vi "Calculate Driving Direction of Tank2_0713.vi"(8 "error in (no error)":errorcluster, 10 "obstacle angles (rad)":dbl[](array[numeric]), 11 "obstacle distances (m)":dbl[](array[numeric])) -> (0 "error out":errorcluster, 3 "steering frame velocity":dbl[](array[numeric]))   [LabVIEW 2012]
doc: "Calculates the velocity vector of the robot required to avoid obstacles, based on the scanned data."
uses:
  <vilib>/robotics/Obstacle Avoidance/Simple Vector Field Histogram/Panic Range.ctl
  <vilib>/Utility/AngleManip/Degrees to Radians (Scalar DBL).vi
  <vilib>/robotics/Obstacle Avoidance/Simple Vector Field Histogram/NI_Robotics_Simple Vector Field Histogram.lvlib
  <vilib>/Utility/AngleManip/NI_AngleManipulation.lvlib
panel:
  out "steering frame velocity 2":dbl[](array[numeric])
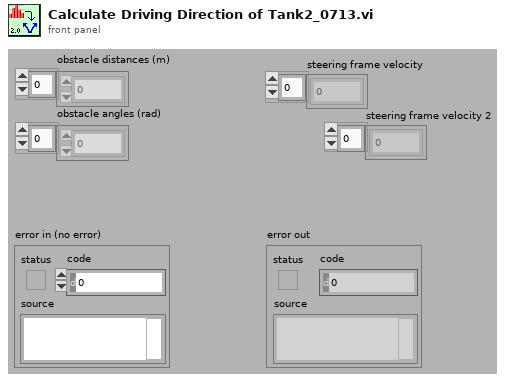
[diagram p1: front panel]
types:
  T1 = typedef "NI_Robotics_Simple Vector Field Histogram.lvlib/Panic Range.ctl" = cluster{"panic threshold distance (0)":dbl, "panic threshold angle (0)":dbl}
  T2 = typedef "NI_Robotics_Simple Vector Field Histogram.lvlib/Obstacle Description.ctl" = cluster{"angle to obstacle":dbl, "distance to obstacle":dbl}
  T3 = typedef "NI_Robotics_Simple Vector Field Histogram.lvlib/Gap Description.ctl" = cluster{"angle to gap":dbl, "size of gap":dbl}
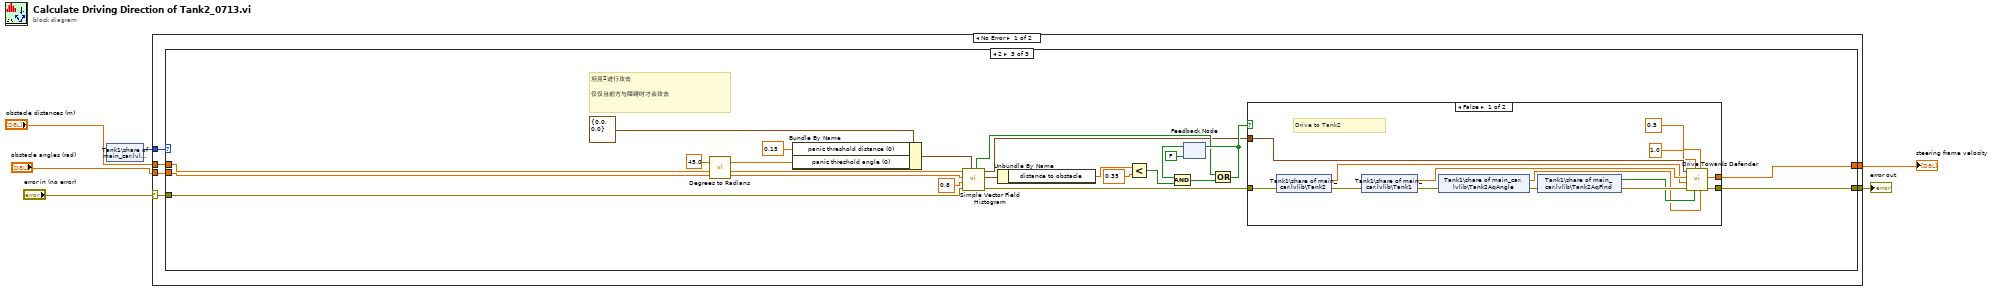
[diagram p0: block diagram]
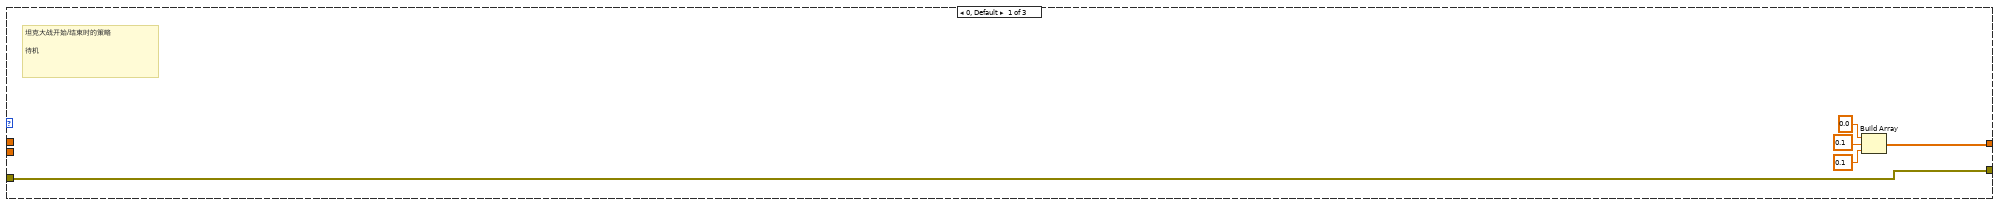
[diagram p2: hidden frame]
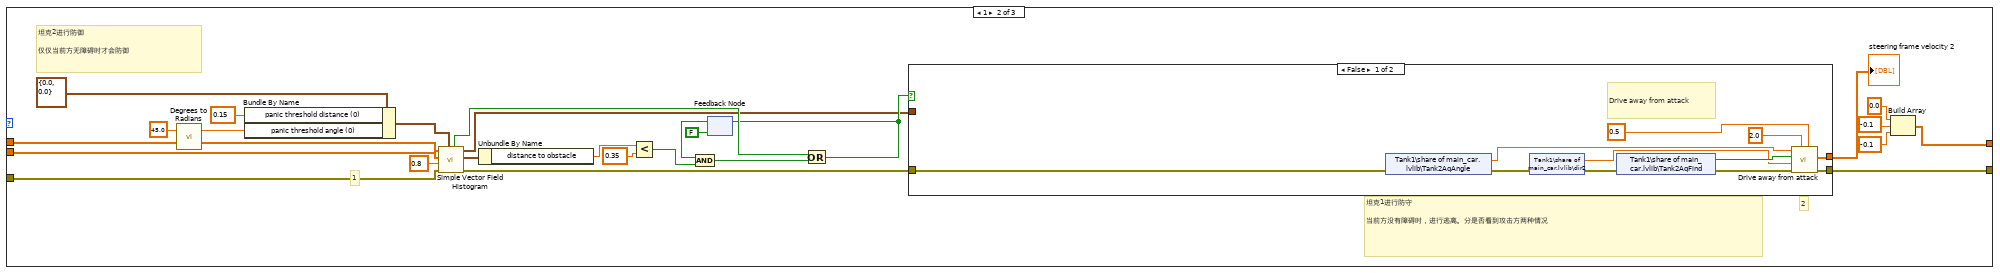
[diagram p3: hidden frame]
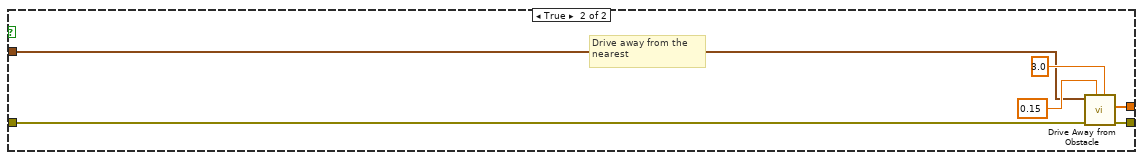
[diagram p4: hidden frame]
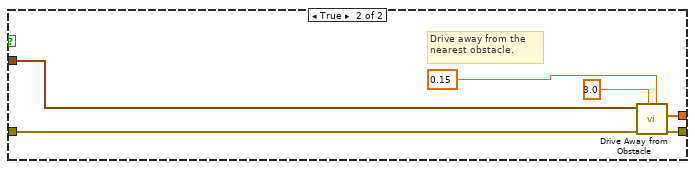
[diagram p5: hidden frame]
diagram:
  n1 = shared-variable "Tank1\\share of main_car.lvlib\\K"() -> (w1:i16)  [unwired: 1 in, 1 out]
  n2 = case shown="No Error" "error in (no error)" {
    selector: "error in (no error)" -> [w12 w103]
    tunnel: [w7 w103] -> w6
    tunnel: "obstacle distances (m)" -> [w11 _]
    tunnel: "obstacle angles (rad)" -> [w10 _]
    tunnel: [w9 _] -> w2
    tunnel: w1 -> [w8 _]
    frame No Error {
      n3 = case shown="2" w8 {
        tunnel: w12 -> [w13 w24 w63]
        tunnel: w11 -> [_ w29 w65]
        tunnel: w10 -> [_ w28 w64]
        tunnel: [w14 w18 w62] -> w9
        tunnel: [w13 w26 w61] -> w7
        frame 0, Default {
          # "坦克大战开始/结束时的策略\n\n待机"
          n4 = Build Array(0.0 ("panic threshold angle (rad)"), 0.1 ("distance threshold (m)"), 0.1 ("distance threshold (m)")) -> (w14:dbl[])
        }
        frame 1 {
          # "2"
          # "坦克1进行防守\n\n当前方没有障碍时，进行逃离。分是否看到攻击方两种情况"
          # "1"
          # "坦克2进行防御\n\n仅仅当前方无障碍时才会防御"
          n5 = call-poly <vilib>:"Degrees to Radians.vi"("angle (deg)"=45.0 ("panic threshold angle (rad)")) -> ("angle (rad)"=w43:dbl)  [unwired: 2 in]
          n6 = Bundle By Name(cluster=T1 {"panic threshold distance (0)"=0.0, "panic threshold angle (0)"=0.0} ("panic range"), "panic threshold distance (0)"=0.15 ("panic threshold distance (m)"), "panic threshold angle (0)"=w43) -> (w32:T1)
          n7 = call <vilib>:"Simple Vector Field Histogram.vi"("panic range"=w32, "error in (no error)"=w24, "distance threshold"=0.8 ("distance threshold (m)"), "direction angles"=w28, "distances"=w29) -> ("error out"=w23:errorcluster, "nearest obstacle"=w34:T2, "largest gap"=w25:T3, "obstacle within panic range"=w39:bool)  [unwired: 2 in, 1 out]
          n8 = Unbundle By Name(w34) -> ("distance to obstacle"=w35:dbl)
          n9 = Less?(x=w35, y=0.35) -> (x < y?=w37:bool)
          n10 = feedback #1(FALSE ("obstacle within panic range")) -> (w38:bool)
          n11 = And(x=w38, y=w37) -> (x .and. y?=w40:bool)
          n12 = Or(x=w39, y=w40) -> (x .or. y?=w27:bool)
          n13 = feedback-in #1(w27) -> ()
          n14 = case shown="False" w27 {
            tunnel: [w54 w60] -> w26
            tunnel: [w50 w55] -> w22
            tunnel: w25 -> [_ w57]
            tunnel: w23 -> [w45 w56]
            frame False {
              # "Drive away from attack"
              n15 = shared-variable "Tank1\\share of main_car.lvlib\\Tank2AqAngle"(error in=w45) -> (w44:dbl, error out=w46:errorcluster)
              n16 = shared-variable "Tank1\\share of main_car.lvlib\\dir2"(error in=w46) -> (w47:dbl, error out=w48:errorcluster)
              n17 = shared-variable "Tank1\\share of main_car.lvlib\\Tank2AqFind"(error in=w48) -> (w49:bool, error out=w51:errorcluster)
              n18 = call "Drive away from attack.vi"("max reverse velocity (m/s)"=0.5 ("max forward velocity (m/s)"), "max angular velocity (rad/s)"=2.0, "error in (no error)"=w51, "dir1"=w47, "find"=w49, "angle"=w44) -> ("error out"=w54:errorcluster, "steering frame velocity"=w50:dbl[])  [unwired: 4 in]
            }
            frame True {
              # "Drive away from the nearest"
              n19 = call "Drive Away from Obstacle.vi"("max reverse velocity (m/s)"=3.0 ("max angular velocity (rad/s)"), "max angular velocity (rad/s)"=0.15 ("max reverse velocity (m/s)"), "error in (no error)"=w56, "gap"=w57) -> ("error out"=w60:errorcluster, "steering frame velocity"=w55:dbl[])  [unwired: 6 in]
            }
          }
          "steering frame velocity 2" <- w22
          n20 = Build Array(0.0 ("panic threshold angle (rad)"), -0.1 ("distance threshold (m)"), -0.1 ("distance threshold (m)")) -> (w18:dbl[])
        }
        frame 2 {
          # "坦克2进行攻击\n\n仅仅当前方与障碍时才会攻击"
          n21 = call-poly <vilib>:"Degrees to Radians.vi"("angle (deg)"=45.0 ("panic threshold angle (rad)")) -> ("angle (rad)"=w82:dbl)  [unwired: 2 in]
          n22 = Bundle By Name(cluster=T1 {"panic threshold distance (0)"=0.0, "panic threshold angle (0)"=0.0} ("panic range"), "panic threshold distance (0)"=0.15 ("panic threshold distance (m)"), "panic threshold angle (0)"=w82) -> (w70:T1)
          n23 = call <vilib>:"Simple Vector Field Histogram.vi"("panic range"=w70, "error in (no error)"=w63, "distance threshold"=0.8 ("distance threshold (m)"), "direction angles"=w64, "distances"=w65) -> ("error out"=w67:errorcluster, "nearest obstacle"=w72:T2, "largest gap"=w66:T3, "obstacle within panic range"=w77:bool)  [unwired: 2 in, 1 out]
          n24 = Unbundle By Name(w72) -> ("distance to obstacle"=w73:dbl)
          n25 = Less?(x=w73, y=0.35) -> (x < y?=w75:bool)
          n26 = feedback #2(FALSE ("obstacle within panic range")) -> (w76:bool)
          n27 = And(x=w76, y=w75) -> (x .and. y?=w78:bool)
          n28 = Or(x=w77, y=w78) -> (x .or. y?=w80:bool)
          n29 = feedback-in #2(w80) -> ()
          n30 = case shown="False" w80 {
            tunnel: w66 -> [w96 w100]
            tunnel: w67 -> [w90 w102]
            tunnel: [w95 w101] -> w61
            tunnel: [w94 w99] -> w62
            frame False {
              # "Drive to Tank2"
              n31 = shared-variable "Tank1\\share of main_car.lvlib\\Tank2"(error in=w90) -> (w83:dbl[], error out=w91:errorcluster)
              n32 = shared-variable "Tank1\\share of main_car.lvlib\\Tank1"(error in=w91) -> (w89:dbl[], error out=w88:errorcluster)
              n33 = shared-variable "Tank1\\share of main_car.lvlib\\Tank2AqAngle"(error in=w88) -> (w84:dbl, error out=w87:errorcluster)
              n34 = shared-variable "Tank1\\share of main_car.lvlib\\Tank2AqFind"(error in=w87) -> (w85:bool, error out=w86:errorcluster)
              n35 = call "Drive Towards Defender.vi"("defencer angle"=w84, "max forward velocity (m/s)"=0.5, "find"=w85, "max angular velocity (rad/s)"=1.0, "error in (no error)"=w86, "attacker"=w83, "defender"=w89, "gap"=w96) -> ("error out"=w95:errorcluster, "steering frame velocity"=w94:dbl[])  [unwired: 2 in]
            }
            frame True {
              # "Drive away from the nearest obstacle."
              n36 = call "Drive Away from Obstacle.vi"("max reverse velocity (m/s)"=0.15, "max angular velocity (rad/s)"=3.0, "error in (no error)"=w102, "gap"=w100) -> ("error out"=w101:errorcluster, "steering frame velocity"=w99:dbl[])  [unwired: 6 in]
            }
          }
        }
      }
    }
    frame Error {
    }
  }
  "error out" <- w6
  "steering frame velocity" <- w2
